vi "Enable Synchronization.vi"(8 "error in (no error)":errorcluster, 9 "Enable Synchronization (T: Enable)":bool=TRUE, 10 "Channel (1:Channel 1)":i32(ring)=1 items=["Channel 1"=1, "Channel 2"=2], 11 "VISA resource name":refnum<visa-resource-name>) -> (0 "error out":errorcluster, 3 "VISA resource name out":refnum<visa-resource-name>)   [LabVIEW 2015, in "SDG X Series.lvlib"]
doc: "Enables or disables synchronization of the Sync output on the back panel to the selected channel's output on the front panel of the instrument.\n\nNote: The sync output can only synchronize with one channel at any given time."
uses:
  <instrlib>/SDG X Series/SDG X Series.lvlib
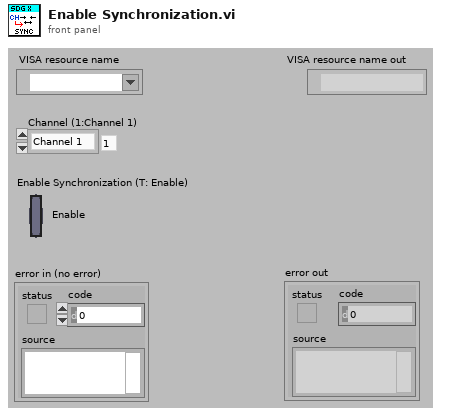
[diagram p1: front panel]
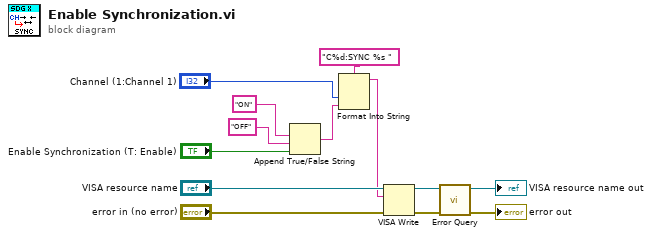
[diagram p0: block diagram]
diagram:
  n1 = Append True/False String(1:"Enable Synchronization (T: Enable)", 2:"OFF" ("true string"), 3:"ON" ("true string")) -> (0:w6:string)  [unwired: 1 in]
  n2 = Format Into String(format string="C%d:SYNC %s ", "Channel (1:Channel 1)", w6) -> (resulting string=w7:string)  [unwired: 2 in, 1 out]
  n3 = VISA Write(VISA resource name="VISA resource name", write buffer=w7, error in (no error)="error in (no error)") -> (VISA resource name out=w3:refnum<visa-resource-name>, error out=w4:errorcluster)  [unwired: 1 out]
  n4 = call <instrlib>:"Error Query.vi"("error in (no error)"=w4, "VISA resource name"=w3) -> ("error out"=→"error out":errorcluster, "VISA resource name out"=→"VISA resource name out":refnum<visa-resource-name>)  [unwired: 6 in, 2 out]
